vi "Wait_until_inaktiv.vi"(4 "error in (no error)":errorcluster caption="Error In", 7 "Pump":T1=enum."P_01") -> (0 "error out":errorcluster caption="Error Out", 3 "Current action finished":bool)   [LabVIEW 2019]
doc: "Waits until the current action has finished.\n\nISM / CS - Jan. '04"
uses:
  Pumpen.ctl
  Inquiring_and_setting_parameters_Reglo_D.ctl
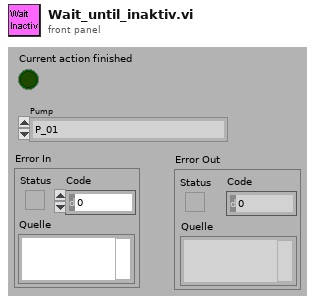
[diagram p1: front panel]
types:
  T1 = typedef "Pumpen.ctl" = enum16{"Pumpe mit Adresse 0 gibt es nicht", "P_01", "P_02", "P_03", "P_04", "P_05", "P_06", "P_07", "P_08"}
  T2 = typedef "Inquiring_and_setting_parameters_Reglo_D.ctl" = enum16{"Current Mode active/inactive ?", "Pump type/Software version/Pump head ?", "Software version ?", "Speed ?", "Speed !", "Default flow rate ?", "Calibrated flow rate ?", "Calibrated flow rate !", "Number of digits after dec.point ?", "Pump tubing inner diameter ?", "Pump tubing inner diameter !", "Dispensing time in 1/10 sec. ?", "Dispensing time in 1/10 sec. !", "Dispensing time in minutes !", "Dispensing time in hours !", "Roller steps for \"MODE DISP - Volume\" ?", "Roller steps for \"MODE DISP - Volume\" !", "Dispensing volume in ml for \"MODE DISP - Volume\" !", "Roller back steps ?", "Roller back steps !", "Pause time in 1/10 sec ?", "Pause time in 1/10 sec. !", "Pause time in minutes !", "Pause time in hours !", "Number of dispensing cycles ?", "Number of dispensing cycles !", "Delivered titration volume ?", "Reset titration volume to 0", "Store application parameters", "Set default values", "Foot switch ?"}
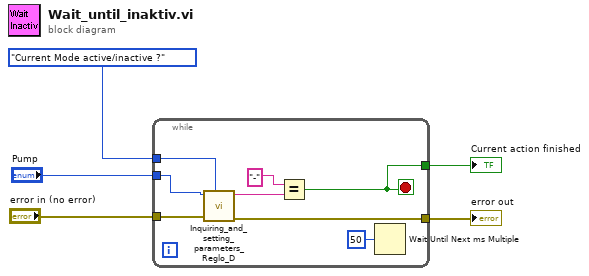
[diagram p0: block diagram]
diagram:
  n1 = while {
    tunnel: "error in (no error)" -> [w13]
    tunnel: [w12] -> w4
    tunnel: "Pump" -> [w11]
    tunnel: Inquiring_and_setting_parameters_Reglo_D."Current Mode active/inactive ?" ("Command") -> [w10]
    tunnel: [w6] -> w1
    stop <- w6 stop-if-true
    n2 = call "Inquiring_and_setting_parameters_Reglo_D.vi"("Command"=w10, "error in (no error)"=w13, "Pumpe"=w11) -> ("error out"=w12:errorcluster, "Answer"=w9:string)  [unwired: 7 in]
    n3 = Equal?(x="-", y=w9) -> (x = y?=w6:bool)
    n4 = Wait Until Next ms Multiple(millisecond multiple=u32 50 ("Vielfache von ms")) -> ()  [unwired: 1 out]
  }
  "error out" <- w4
  "Current action finished" <- w1
